vi "FTW-ProjectItemManager-TransactionQueueFlush.vi"(0 "Project Item Manager":refnum<class "FTW-ProjectItemManager.lvclass">, 11 "error in":errorcluster) -> (4 "Project Item Manager out":refnum<class "FTW-ProjectItemManager.lvclass">, 6 "Remove Transaction Tags Removed":string[](array[string]), 8 "Write Transaction Tags Removed":string[](array[string]), 10 "Write Transaction Tag Values Removed":variant[](array[variant]), 15 "error out":errorcluster)   [LabVIEW 2012, in "FTW-ProjectItemManager.lvclass"]
doc: "This method removes all Persistent Properties within the Property Bag that are waiting to be written to the Project Item."
uses:
  FTW-ProjectItemManager.lvclass
  FTW-ProjectItemManager.lvclass/FTW-ProjectItemManager.ctl
panel:
  # "Inputs"
  # "Outputs"
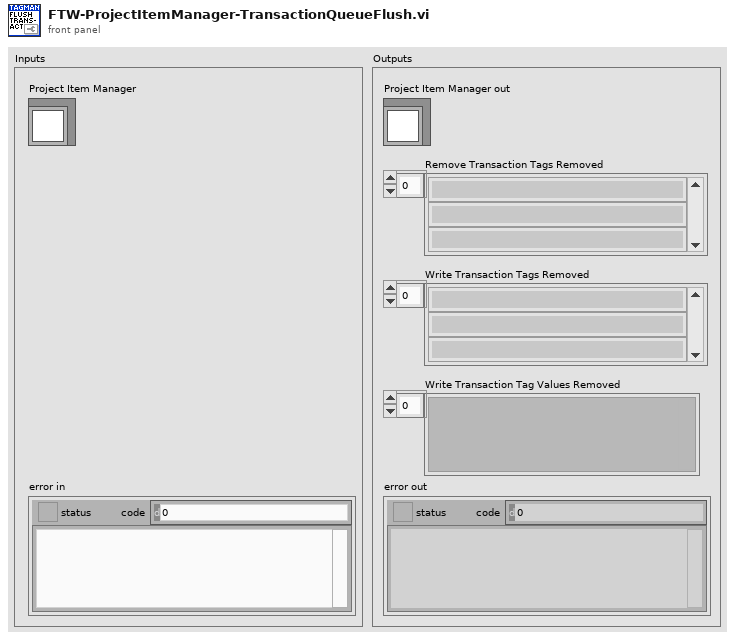
[diagram p1: front panel]
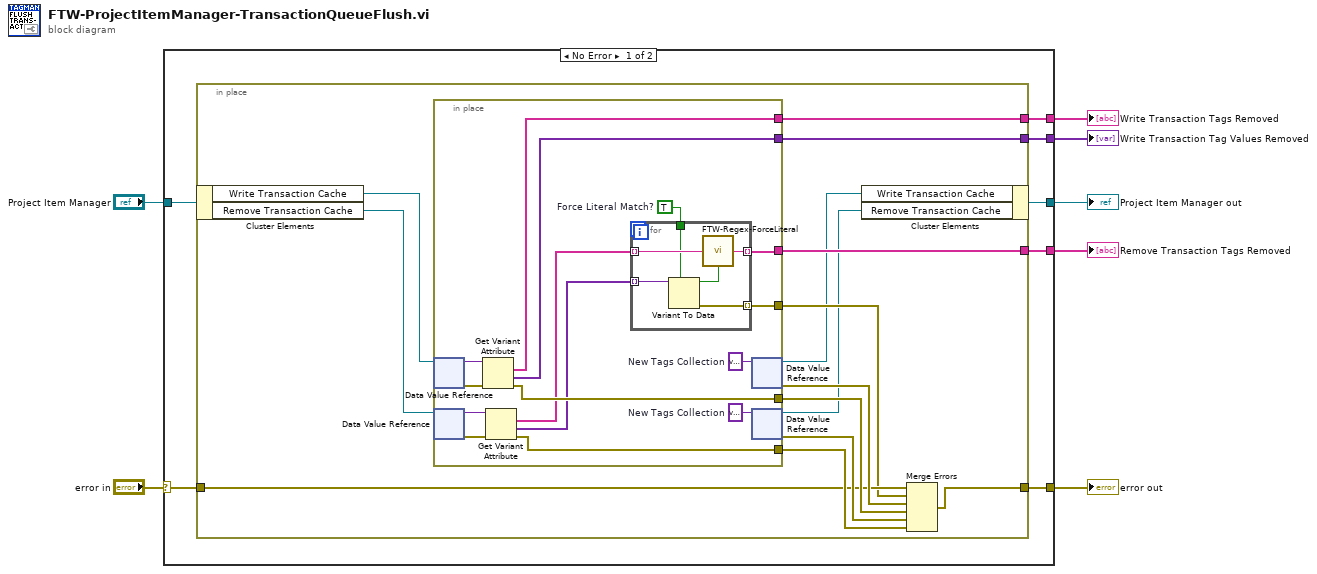
[diagram p0: block diagram]
diagram:
  n1 = case shown="No Error" "error in" {
    selector: "error in" -> [w12 w51]
    tunnel: [w11 w51] -> w7
    tunnel: [w13 w50] -> w5
    tunnel: "Project Item Manager" -> [w14 w50]
    tunnel: [w10 _] -> w3
    tunnel: [w9 _] -> w2
    tunnel: [w8 _] -> w1
    frame No Error {
      n2 = in-place {
        in-place-border: w12 -> [w18]
        in-place-border: [w25] -> w11
        in-place-border: [w27] -> w10
        in-place-border: [w24] -> w9
        in-place-border: [w19] -> w8
        n3 = in-place-cluster #1(w14) -> ("Write Transaction Cache"=w28:refnum<data-value>, "Remove Transaction Cache"=w22:refnum<data-value>)
        n4 = in-place {
          in-place-border: [w40] -> w27
          in-place-border: [w39] -> w24
          in-place-border: [w38] -> w23
          in-place-border: [w34] -> w20
          in-place-border: [w31] -> w19
          in-place-border: [w29] -> w17
          w30 = TRUE  # Force Literal Match?
          w35 = variant  # New Tags Collection
          w41 = variant  # New Tags Collection
          n5 = in-place-dvr #2(w28) -> (w43:variant, w42:errorcluster)
          n6 = in-place-dvr #3(w22) -> (w37:variant, w36:errorcluster)
          n7 = Get Variant Attribute(Variant=w43, error in=w42) -> (names=w40:string[], values=w39:variant[], error out=w38:errorcluster)  [unwired: 2 in, 1 out]
          n8 = Get Variant Attribute(Variant=w37, error in=w36) -> (names=w32:string[], values=w33:variant[], error out=w34:errorcluster)  [unwired: 2 in, 1 out]
          n9 = for {
            tunnel: w33 -> [w49] mode=indexing
            tunnel: w32 -> [w48] mode=indexing
            tunnel: [w47] -> w31 mode=indexing
            tunnel: [w46] -> w29 mode=indexing
            tunnel: w30 -> [w44]
            n10 = Variant To Data(type=w44, Variant=w49) -> (data=w45:bool, error out=w46:errorcluster)  [unwired: 1 in]
            n11 = call "FTW-Regex-ForceLiteral.vi"("Input"=w48, "Force Literal Match?"=w45) -> ("Output"=w47:string)
          }
          n12 = in-place-dvr #2(w41) -> (w15:refnum<data-value>, w26:errorcluster)
          n13 = in-place-dvr #3(w35) -> (w16:refnum<data-value>, w21:errorcluster)
        }
        n14 = in-place-cluster #1("Write Transaction Cache"=w15, "Remove Transaction Cache"=w16) -> (w13:refnum<class "FTW-ProjectItemManager.lvclass">)
        n15 = Merge Errors(w18, w17, w26, w23, w21, w20) -> (w25:errorcluster)
      }
    }
    frame Error {
    }
  }
  "error out" <- w7
  "Project Item Manager out" <- w5
  "Write Transaction Tags Removed" <- w3
  "Write Transaction Tag Values Removed" <- w2
  "Remove Transaction Tags Removed" <- w1
